vi "BRig_Host__Loop_Consumer_RunState__loadData_subunit1.vi"(10 "input_data":u16[](array[numeric]), 11 "input_name":string="dataExp") -> (2 "output_data":u16[](array[numeric]), 3 "output_data":bool)   [LabVIEW 2014]
uses:
  <vilib>/Utility/file.llb/Read From Spreadsheet File (I64).vi
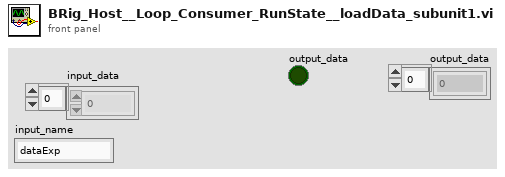
[diagram p1: front panel]
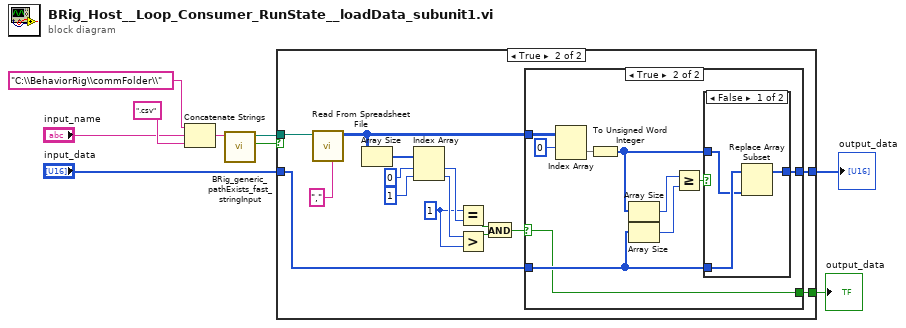
[diagram p0: block diagram]
diagram:
  n1 = Concatenate Strings("C:\\BehaviorRig\\commFolder\\", "input_name", ".csv" ("string")) -> (w4:string)
  n2 = call "BRig_generic_pathExists_fast_stringInput.vi"("input_filePath"=w4) -> ("output_Iexist"=w2:bool, "output_filePath"=w3:path)  [unwired: 8 in, 1 out]
  n3 = case shown="True" w2 {
    tunnel: w3 -> [_ w25]
    tunnel: "input_data" -> [w10 w19]
    tunnel: [w10 w18] -> w6
    tunnel: [_ w11] -> w1
    frame False {
    }
    frame True {
      w13 = 1 ("x")
      n4 = call-poly <vilib>:"Read From Spreadsheet File.vi"("delimiter (\\t)"="," ("delimiter (\\t)"), "file path (dialog if empty)"=w25) -> ("all rows"=w17:i64[][])  [unwired: 5 in, 4 out]
      n5 = Array Size(array=w17) -> (size(s)=w23:i32[])
      n6 = Index Array(array=w23, index #1=0 ("index"), index #2=1 ("index")) -> (element #1=w16:i32, element #2=w14:i32)
      n7 = Equal?(x=w13, y=w16) -> (x = y?=w15:bool)
      n8 = Greater?(x=w14, y=w13) -> (0:w12:bool)
      n9 = And(x=w15, y=w12) -> (x .and. y?=w20:bool)
      n10 = case shown="True" w20 {
        selector: w20 -> [_ w27]
        tunnel: w19 -> [w26 w28]
        tunnel: [w26 w29] -> w18
        tunnel: w17 -> [_ w36]
        tunnel: [_ w27] -> w11
        frame False {
        }
        frame True {
          n11 = Index Array(array=w36, index (row)=0) -> (element=w34:i64[])  [unwired: 1 in]
          n12 = To Unsigned Word Integer(number=w34) -> (unsigned 16bit integer=w30:u16[])
          n13 = Array Size(array=w30) -> (size(s)=w33:i32)
          n14 = Array Size(array=w28) -> (size(s)=w32:i32)
          n15 = Greater Or Equal?(x=w33, y=w32) -> (x >= y?=w31:bool)
          n16 = case shown="False" w31 {
            tunnel: w30 -> [w38 w40]
            tunnel: [w37 w40] -> w29
            tunnel: w28 -> [w39 _]
            frame False {
              n17 = Replace Array Subset(array=w39, new element=w38) -> (w37:u16[])  [unwired: 1 in]
            }
            frame True {
            }
          }
        }
      }
    }
  }
  "output_data" <- w6
  "output_data" <- w1
